vi "String to Number.vi"(11 "Decimal String":string) -> (3 "Decimal Number":i32)   [LabVIEW 2021]
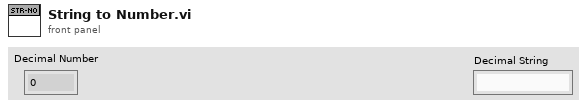
[diagram p1: front panel]
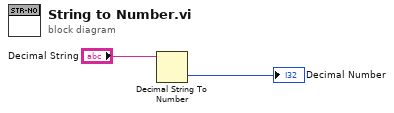
[diagram p0: block diagram]
diagram:
  n1 = Decimal String To Number(string="Decimal String") -> (number=→"Decimal Number":i32)  [unwired: 2 in, 1 out]
